vi "LRU Cache.vi"   [LabVIEW 2019, in "23.lvlib"]
uses:
  23.lvlib
types:
  T1 = map{cluster{"Hallway":string[], "Rooms":string[][]}, u64}
  T2 = cluster{"Stop":bool, "Check":bool, "Key":cluster{"Hallway":string[], "Rooms":string[][]}, "Value":u64, "Check Notifier":refnum<notifier>}
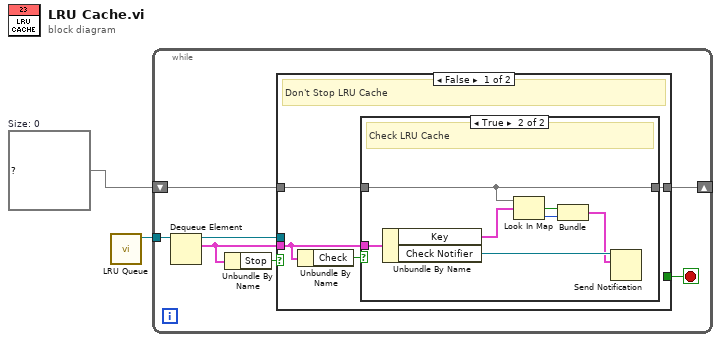
[diagram p0: block diagram]
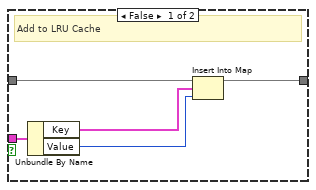
[diagram p2: hidden frame]
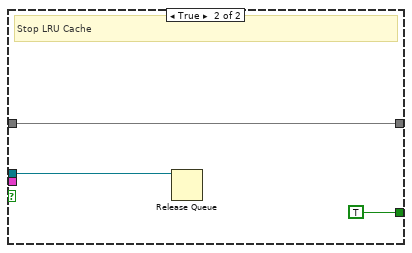
[diagram p3: hidden frame]
diagram:
  w1 = T1 {}  # Size: 0
  n1 = call "LRU Queue.vi"() -> ("LRU Queue"=w2:refnum<queue>)  [unwired: 11 in]
  n2 = while {
    shift-right: [w4] -> _
    shift-left: w1 -> [w9]
    tunnel: w2 -> [w8]
    stop <- w3 stop-if-true
    n3 = Dequeue Element(queue=w8) -> (queue out=w6:refnum<queue>, element=w5:T2)  [unwired: 2 in, 2 out]
    n4 = Unbundle By Name(w5) -> ("Stop"=w7:bool)
    n5 = case shown="False" w7 {
      tunnel: w9 -> [w11 w27]
      tunnel: w6 -> [_ w28]
      tunnel: w5 -> [w12 _]
      tunnel: [w10 w27] -> w4
      tunnel: [_ TRUE] -> w3
      frame False {
        # "Don't Stop LRU Cache"
        n6 = Unbundle By Name(w12) -> ("Check"=w13:bool)
        n7 = case shown="True" w13 {
          tunnel: w12 -> [w18 w24]
          tunnel: w11 -> [w16 w25]
          tunnel: [w17 w25] -> w10
          frame False {
            # "Add to LRU Cache"
            n8 = Unbundle By Name(w18) -> ("Key"=w15:cluster{"Hallway":string[], "Rooms":string[][]}, "Value"=w14:u64)
            n9 = Insert Into Map(map in=w16, key=w15, value=w14) -> (map out=w17:T1)  [unwired: 2 out]
          }
          frame True {
            # "Check LRU Cache"
            n10 = Unbundle By Name(w24) -> ("Key"=w23:cluster{"Hallway":string[], "Rooms":string[][]}, "Check Notifier"=w20:refnum<notifier>)
            n11 = Look In Map(map=w25, key=w23) -> (key not found?=w22:bool, value=w21:u64)  [unwired: 1 in]
            n12 = Bundle("key not found?"=w22, "Value"=w21) -> (w19:cluster{"key not found?":bool, "Value":u64})  [unwired: 1 in]
            n13 = Send Notification(notification=w19, notifier=w20) -> ()  [unwired: 1 in, 2 out]
          }
        }
      }
      frame True {
        # "Stop LRU Cache"
        n14 = Release Queue(queue=w28) -> ()  [unwired: 2 in, 3 out]
      }
    }
  }
